vi "Transceiver Interface.Destroy.vi"(8 "error in (no error)":errorcluster, 11 "Transceiver Interface in":refnum<class "Transceiver Interface.lvclass">) -> (0 "error out":errorcluster)   [LabVIEW 2017, in "DSF.Engine.lvlib" / "Transceiver Interface.lvclass"]
uses:
  Transceiver Interface.lvclass
  C:/Git/DSF/dsf core/Source/Engine/Classes/Interface/Interface.lvclass
  Interface.lvclass
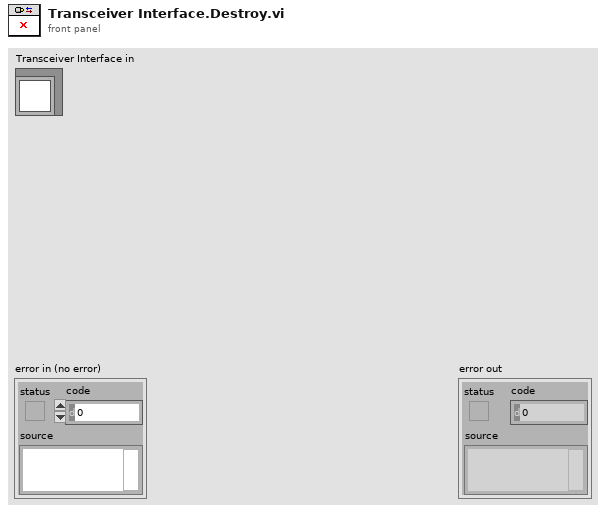
[diagram p1: front panel]
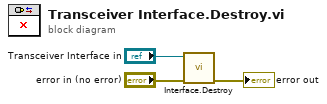
[diagram p0: block diagram]
diagram:
  n1 = call "Interface.Destroy.vi"("error in (no error)"="error in (no error)", "Interface in"="Transceiver Interface in") -> ("error out"=→"error out":errorcluster)  [unwired: 7 in, 2 out]
